vi "Configure Impedance Compensation.vi"(8 "error in (no error)":errorcluster, 10 "Impedance Compensation (0: None)":i32(ring) items=["None", "2-wire", "4-wire"], 11 "VISA resource name":refnum<visa-resource-name>) -> (0 "error out":errorcluster, 3 "VISA resource name out":refnum<visa-resource-name>)   [LabVIEW 2012, in "Fluke 5080.lvlib"]
doc: "Sets whether or not activates (2-wire or 4-wire) impedance compensation."
uses:
  <instrlib>/Fluke 5080/Fluke 5080.lvlib
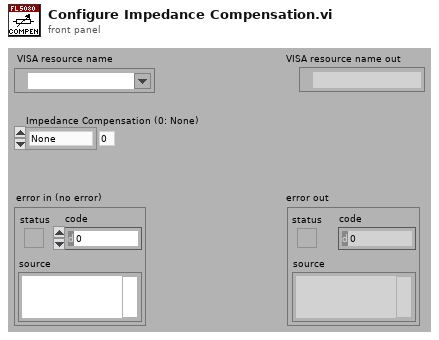
[diagram p1: front panel]
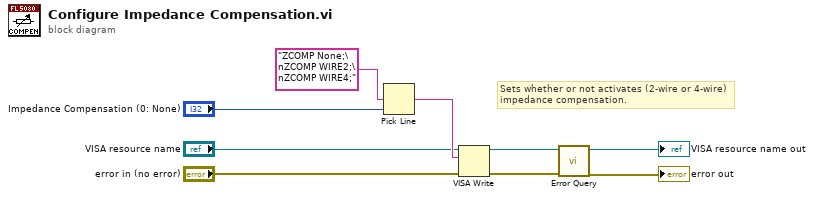
[diagram p0: block diagram]
diagram:
  # "Sets whether or not activates (2-wire or 4-wire) \nimpedance compensation."
  n1 = Pick Line(multi-line string="ZCOMP None;\nZCOMP WIRE2;\nZCOMP WIRE4;", line index="Impedance Compensation (0: None)") -> (output string=w7:string)  [unwired: 1 out]
  n2 = VISA Write(VISA resource name="VISA resource name", write buffer=w7, error in (no error)="error in (no error)") -> (VISA resource name out=w4:refnum<visa-resource-name>, error out=w3:errorcluster)  [unwired: 1 out]
  n3 = call <instrlib>:"Error Query.vi"("error in (no error)"=w3, "VISA resource name"=w4) -> ("error out"=→"error out":errorcluster, "VISA resource name out"=→"VISA resource name out":refnum<visa-resource-name>)  [unwired: 8 out]
